vi "ValudateHTTPURI.vi"(0 "HTTP URI":string="http://hostname.domain:80/resource/name") -> (4 "HTTP URI Out":string="ws://hostname.domain:80/resource/name", 8 "Relative":bool, 15 "Valid HTTP URI":bool)   [LabVIEW 2017, in "LV WebSockets.lvlib"]
uses:
  LV WebSockets.lvlib
  <vilib>/regexp/Match Regular Expression.xnode
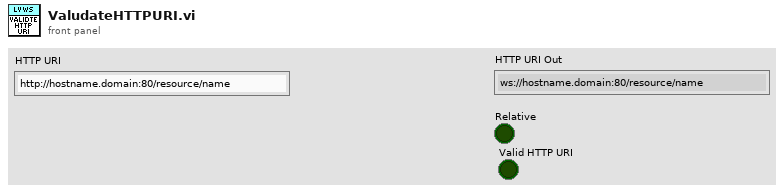
[diagram p1: front panel]
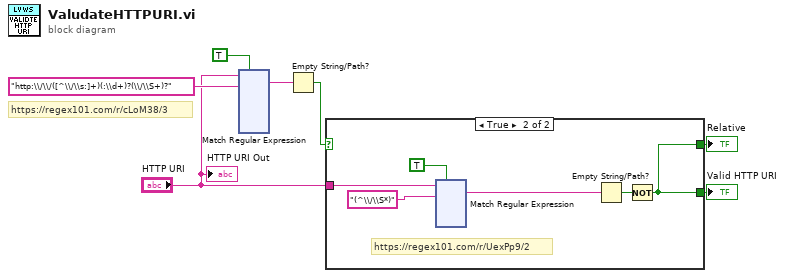
[diagram p0: block diagram]
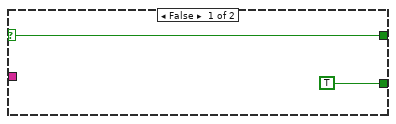
[diagram p2: hidden frame]
diagram:
  # "https://regex101.com/r/cLoM38/3"
  n1 = xnode "Match Regular Expression"("input string"="HTTP URI", "regular expression"="http:\\/\\/([^\\/\\s:]+)(:\\d+)?(\\/\\S+)?", "ignore case? (F)"=TRUE) -> ("whole match"=w7:string)  [unwired: 3 in, 7 out]
  n2 = Empty String/Path?(string/path=w7) -> (empty?=w5:bool)
  n3 = case shown="True" w5 {
    selector: w5 -> [w9 _]
    tunnel: "HTTP URI" -> [_ w14]
    tunnel: [w9 w10] -> w2
    tunnel: [TRUE w10] -> w1
    frame False {
    }
    frame True {
      # "https://regex101.com/r/UexPp9/2"
      n4 = xnode "Match Regular Expression"("input string"=w14, "regular expression"="(^\\/\\S*)", "ignore case? (F)"=TRUE) -> ("whole match"=w12:string)  [unwired: 3 in, 5 out]
      n5 = Empty String/Path?(string/path=w12) -> (empty?=w11:bool)
      n6 = Not(x=w11) -> (.not. x?=w10:bool)
    }
  }
  "Relative" <- w2
  "Valid HTTP URI" <- w1
  "HTTP URI Out" <- "HTTP URI"
